vi "Cal Validation.vi"(0 "Path In":path, 5 "Probe Mic Gain (dB)":dbl, 7 "Cal Mic Gain (dB)":dbl, 9 "Cal Mic Sens (dB)":dbl, 11 "Ear":T2) -> ()   [LabVIEW 2020]
uses:
  Utility VIs/Type Defs/Left-Right ring.ctl
  Type Defs/Cal-Smoothing Parameters.ctl
  Type Defs/CalVal-Params.ctl
panel:
  out "Smooth Params":T1={"Method"=enum."Loess", "MA"={"Iterations"=100, "Length"=3}, "Loess"={"Length"=21, "Type"=enum."Quadratic", "Robust"=TRUE}} {"Loess"."Length" min=1 step=1; "MA"."Length" min=1 step=1; "MA"."Iterations" min=1 step=1}
  in  "Save Button":bool
  out "df (Hz)":dbl
  out "Fs (Hz)":dbl
  out "Frequency (Hz)":dbl
  out "Test Freqs":dbl[](array[numeric])
  out "Error Graph":T3(graph)
  out "Mag Graph":T3(graph)
  out "exit signal":bool
  out "Path":path
  out "running":bool
  in  "Exit":bool
  in  "Go":bool
  out "Abort":bool
  in  "Stop":bool
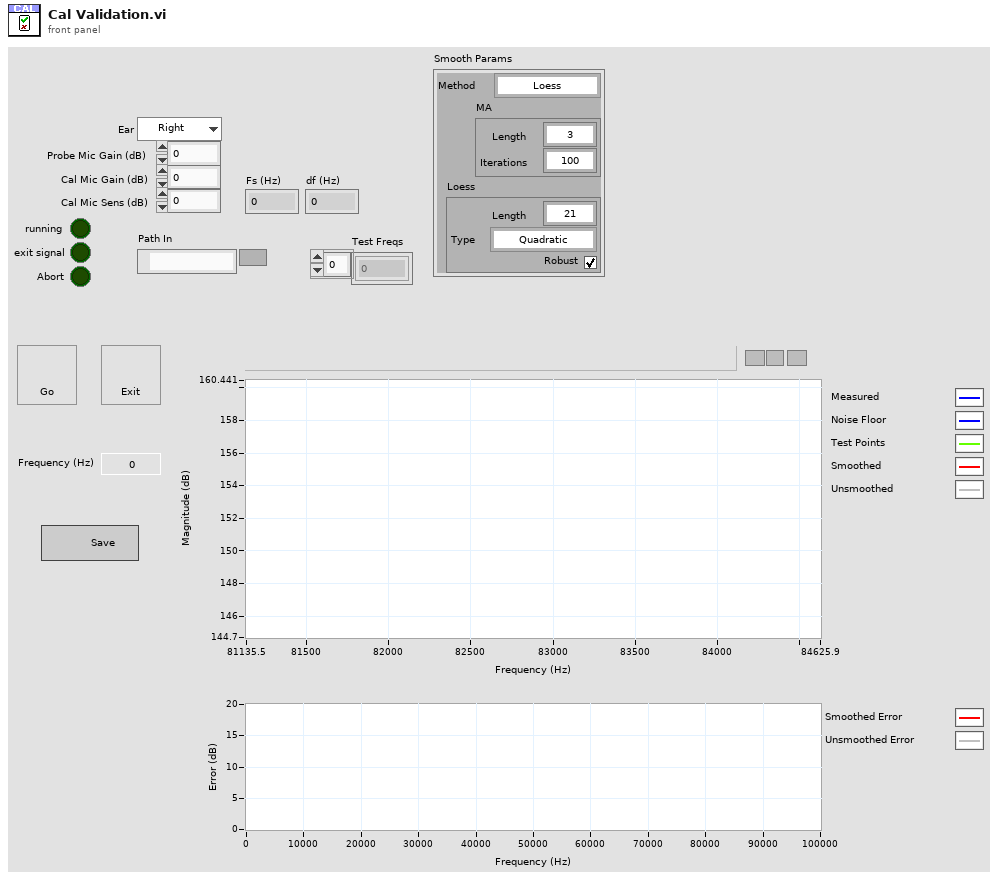
[diagram p1: front panel]
types:
  T1 = typedef "Cal-Smoothing Parameters.ctl" = cluster{"Method":enum16{"None", "Moving average", "Loess"}, "MA":cluster{"Iterations":i32, "Length":i32}, "Loess":cluster{"Length":i32, "Type":enum16{"Linear", "Quadratic"}, "Robust":bool}}
  T2 = typedef "Left-Right ring.ctl" = enum16{"Right", "Left"}
  T3 = cluster{"Frequency (Hz)":dbl[], "Unsmoothed Mag":dbl[]}[]
  T4 = cluster{"Freq (Hz)":dbl, "Val (dB SPL/V)":dbl, "Noise Floor":dbl}
  T5 = typedef "CalVal-Params.ctl" = cluster{"Fs (Hz)":dbl, "Duration (s)":dbl, "Ear":T2, "Probe Mic Gain (dB)":dbl, "Cal Mic Gain (dB)":dbl, "Cal Mic Sens (dB)":dbl, "AO Channels":i32[], "NPts/buffer":i32, "Probe-Cal Indices":i32[]}
  T6 = enum8{"Enabled", "Disabled", "Disabled and Grayed Out"}
  T7 = cluster{"Frequency (Hz)":dbl[], "Unsmoothed Mag":dbl[]}
  T8 = cluster{"Length":i32, "Type":enum16{"Linear", "Quadratic"}, "Robust":bool}
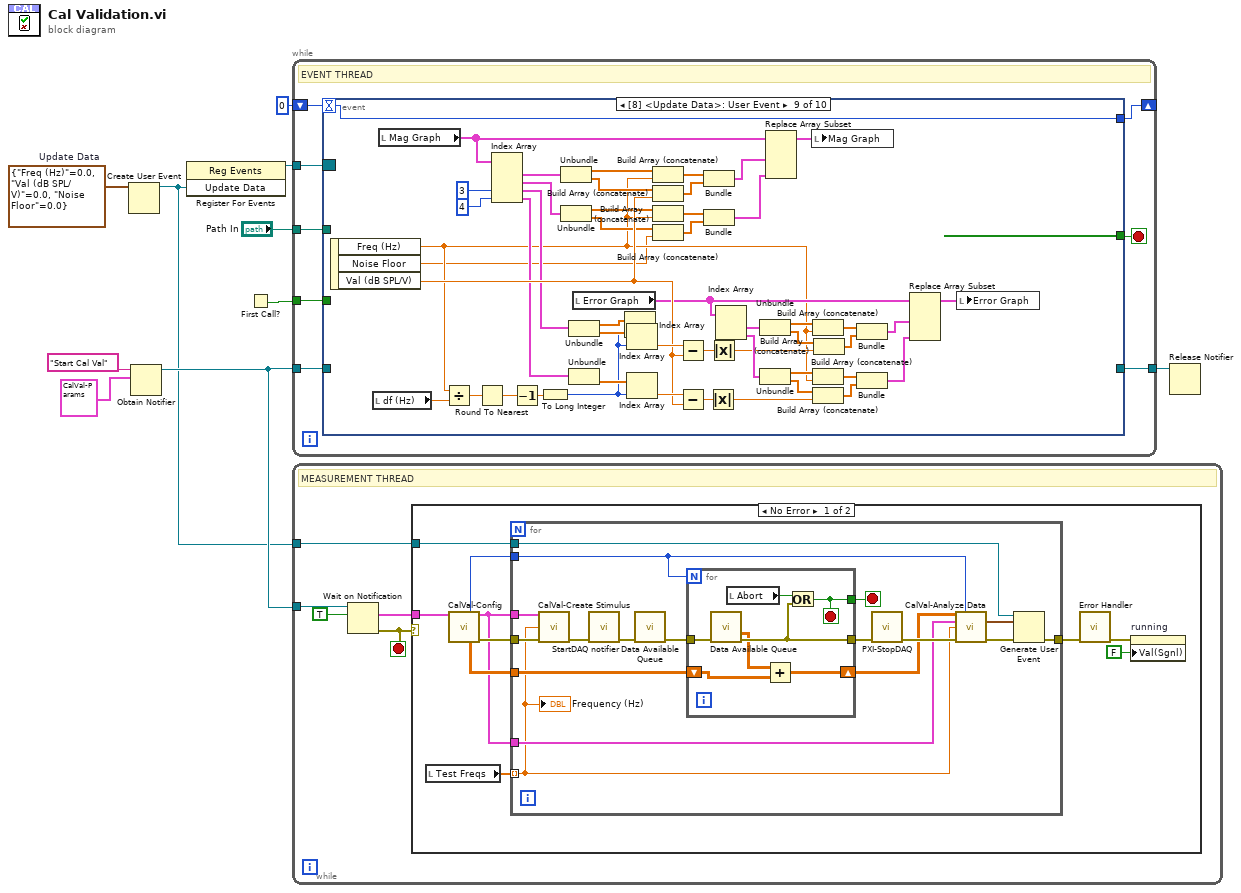
[diagram p0: block diagram]
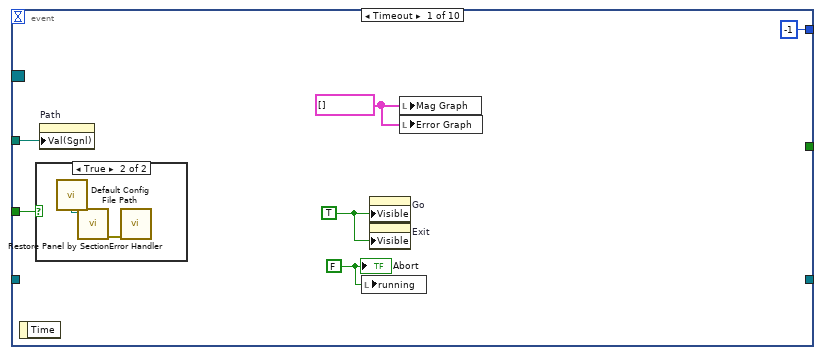
[diagram p3: hidden frame]
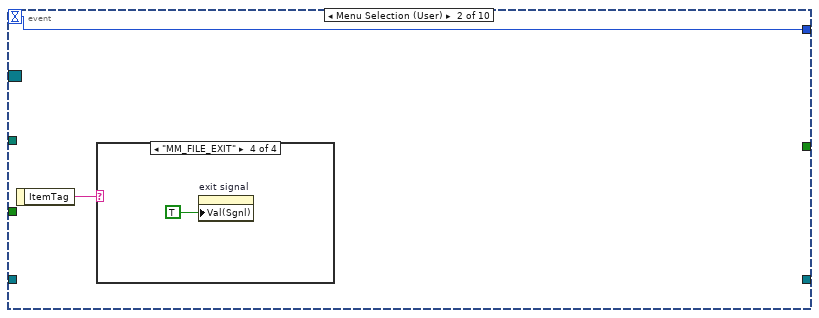
[diagram p5: hidden frame]
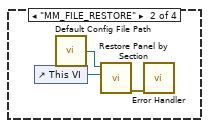
[diagram p7: hidden frame]
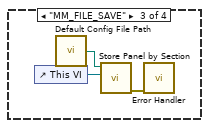
[diagram p8: hidden frame]
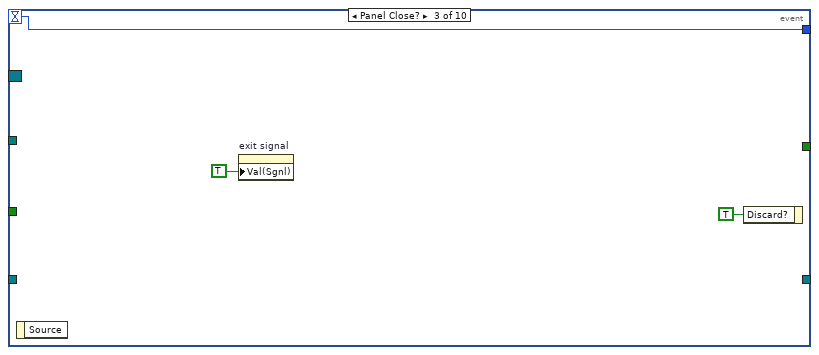
[diagram p9: hidden frame]
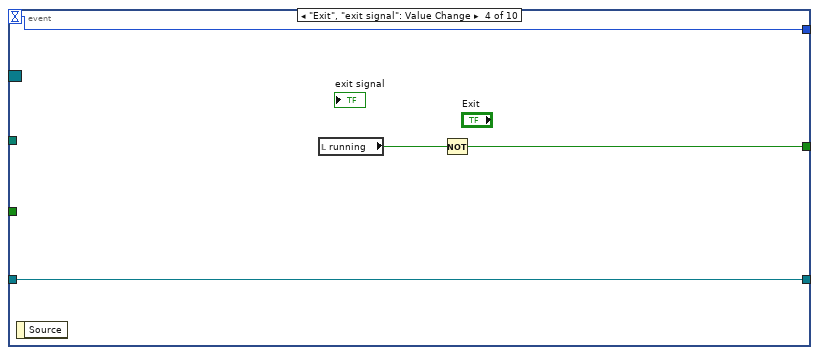
[diagram p10: hidden frame]
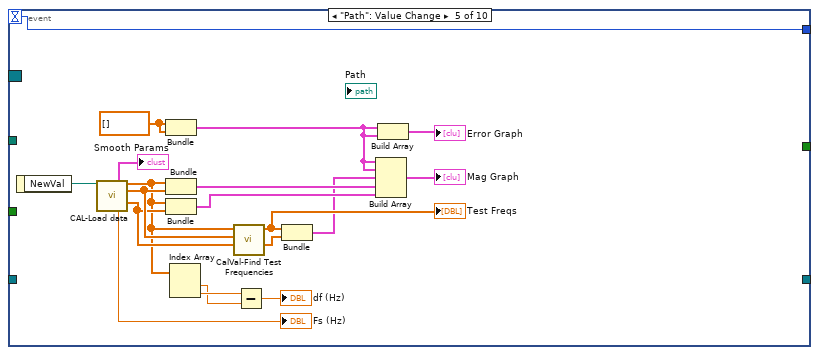
[diagram p11: hidden frame]
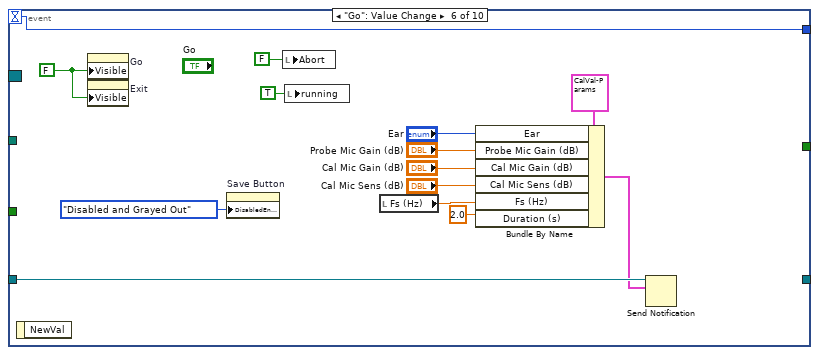
[diagram p12: hidden frame]
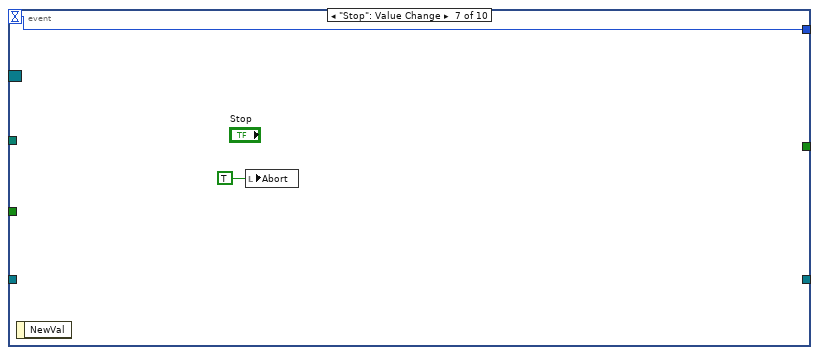
[diagram p13: hidden frame]
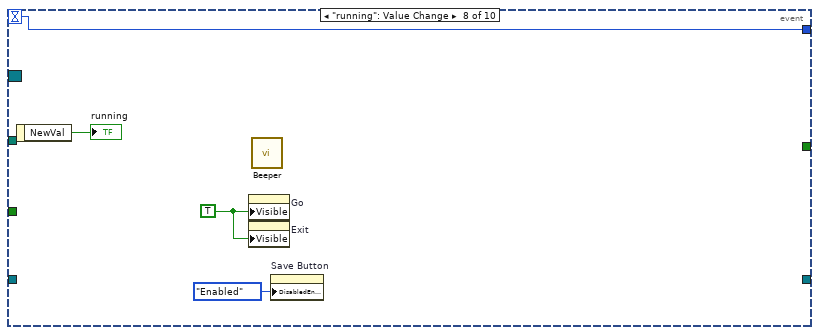
[diagram p14: hidden frame]
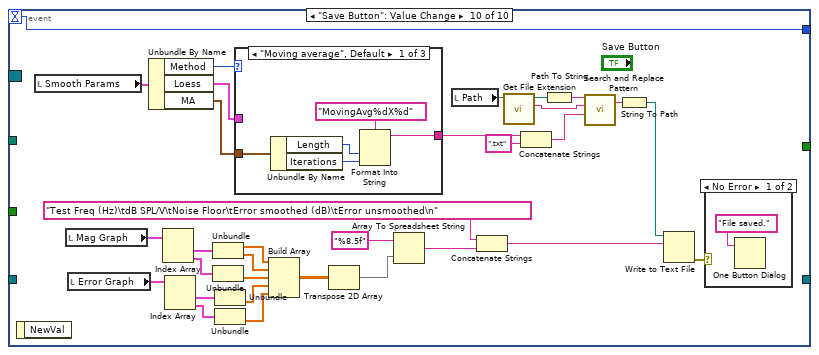
[diagram p15: hidden frame]
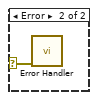
[diagram p16: hidden frame]
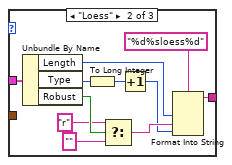
[diagram p17: hidden frame]
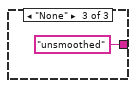
[diagram p18: hidden frame]
diagram:
  w2 = T4 {"Freq (Hz)"=0.0, "Val (dB SPL/V)"=0.0, "Noise Floor"=0.0}  # Update Data
  n1 = Create User Event(user event datatype=w2) -> (user event=w1:refnum<user-event>)  [unwired: 1 in, 1 out]
  n2 = Obtain Notifier(name (unnamed)="Start Cal Val", notification data type=T5 {"Fs (Hz)"=0.0, "Duration (s)"=0.0, "Ear"=enum."Right", "Probe Mic Gain (dB)"=0.0, "Cal Mic Gain (dB)"=0.0, "Cal Mic Sens (dB)"=0.0, "AO Channels"=[], "NPts/buffer"=0, "Probe-Cal Indices"=[]} ("Params")) -> (notifier out=w10:refnum<notifier>)  [unwired: 2 in, 2 out]
  n3 = register-events(w1) -> (reference out=w3:refnum<event-registration>)  [unwired: 2 in, 1 out]
  n4 = First Call?() -> (First Call?: T/F=w6:bool)
  n5 = while {
    tunnel: w10 -> [w18]
    tunnel: [w16] -> w9
    shift-right: [w14] -> _
    shift-left: 0 -> [w15]
    tunnel: w6 -> [w13]
    tunnel: "Path In" -> [w12]
    tunnel: w3 -> [w11]
    stop <- w17 stop-if-true
    # "EVENT THREAD"
    n6 = event shown="[8] <Update Data>: User Event" {
      selector: w11 -> [_ _ _ _ _ _ _ _ _ _]
      dyn-events: _ -> [_ _ _ _ _ _ _ _ _ _]
      timeout: w15 -> [_ w27 w38 w41 w61 w73 w76 w81 w131 w163]
      tunnel: w18 -> [_ _ _ w42 _ w75 _ _ _ _]
      tunnel: [_ _ _ w39 _ _ _ _ _ _] -> w17
      tunnel: [_ _ _ w42 _ _ _ _ _ _] -> w16
      tunnel: [-1 w27 w38 w41 w61 w73 w76 w81 w131 w163] -> w14
      tunnel: w13 -> [w22 _ _ _ _ _ _ _ _ _]
      tunnel: w12 -> [w19 _ _ _ _ _ _ _ _ _]
      event Timeout {
        w20 = T3 [] ("Mag Graph")
        w21 = TRUE ("Visible")
        w23 = FALSE ("Abort")
        n7 = event-data() -> ()  [unwired: 1 in, 1 out]
        n8 = case shown="True" w22 {
          frame False {
          }
          frame True {
            n9 = call "Default Config File Path.vi"() -> ("Default config file name"=w25:path)
            n10 = call "Restore Panel by Section.vi"("Path (dialog)"=w25) -> ("Error Out"=w26:errorcluster)  [unwired: 10 in]
            n11 = call "Error Handler.vi"("error in (no error)"=w26) -> ()  [unwired: 13 in, 2 out]
          }
        }
        n12 = property on="Path" class="Path"("Val(Sgnl)"=w19) -> ()  [unwired: 2 in, 2 out]
        n13 = local write "running"(w23) -> ()
        n14 = property on="Go" class="Bool"("Visible"=w21) -> ()  [unwired: 2 in, 2 out]
        n15 = property on="Exit" class="Bool"("Visible"=w21) -> ()  [unwired: 2 in, 2 out]
        n16 = local write "Mag Graph"(w20) -> ()
        n17 = local write "Error Graph"(w20) -> ()
        "Abort" <- w23
      }
      event Menu Selection (User) {
        n18 = event-data() -> ("ItemTag"=w28:string)  [unwired: 1 in]
        n19 = case shown="\"MM_FILE_EXIT\"" w28 {
          frame "False", Default {
          }
          frame "MM_FILE_RESTORE" {
            n20 = control-ref of="This VI"() -> (w30:refnum<vi>)
            n21 = call "Default Config File Path.vi"() -> ("Default config file name"=w29:path)
            n22 = call "Restore Panel by Section.vi"("VI reference"=w30, "Path (dialog)"=w29) -> ("Error Out"=w31:errorcluster)  [unwired: 9 in]
            n23 = call "Error Handler.vi"("error in (no error)"=w31) -> ()  [unwired: 13 in, 2 out]
          }
          frame "MM_FILE_SAVE" {
            n24 = control-ref of="This VI"() -> (w33:refnum<vi>)
            n25 = call "Default Config File Path.vi"() -> ("Default config file name"=w32:path)
            n26 = call "Store Panel by Section.vi"("VI reference"=w33, "Path (dialog)"=w32) -> ("Error Out"=w34:errorcluster)  [unwired: 9 in]
            n27 = call "Error Handler.vi"("error in (no error)"=w34) -> ()  [unwired: 13 in, 2 out]
          }
          frame "MM_FILE_EXIT" {
            n28 = property on="exit signal" class="Bool (strict)"("Val(Sgnl)"=TRUE ("Value (Signaling)")) -> ()  [unwired: 2 in, 2 out]
          }
        }
      }
      event Panel Close? {
        n29 = event-data() -> ()  [unwired: 1 in, 1 out]
        n30 = property on="exit signal" class="Bool (strict)"("Val(Sgnl)"=TRUE ("Value (Signaling)")) -> ()  [unwired: 2 in, 2 out]
        n31 = event-data("Discard?"=TRUE) -> ()  [unwired: 1 in, 1 out]
      }
      event "Exit", "exit signal": Value Change {
        n32 = event-data() -> ()  [unwired: 1 in, 1 out]
        n33 = local read "running"() -> (w40:bool)
        n34 = Not(x=w40) -> (.not. x?=w39:bool)
      }
      event "Path": Value Change {
        w57 = dbl[] []
        n35 = event-data() -> ("NewVal"=w60:path)  [unwired: 1 in]
        n36 = call "CAL-Load data.vi"("user path"=w60) -> ("Smooth Params"=→"Smooth Params":T1, "Frequency (Hz)"=w46:dbl[], "Mag"=w56:dbl[], "Unsmoothed Mag"=w55:dbl[], "Fs (Hz)"=→"Fs (Hz)":dbl)  [unwired: 7 in, 3 out]
        n37 = Bundle(w57, w57) -> (w48:cluster{dbl[], dbl[]})  [unwired: 1 in]
        n38 = Bundle("Frequency (Hz)"=w46, "Mag"=w56) -> (w59:cluster{"Frequency (Hz)":dbl[], "Mag":dbl[]})  [unwired: 1 in]
        n39 = Bundle("Frequency (Hz)"=w46, "Unsmoothed Mag"=w55) -> (w58:T7)  [unwired: 1 in]
        n40 = Index Array(array=w46) -> (element #1=w44:dbl, element #2=w45:dbl)  [unwired: 2 in]
        n41 = call "CalVal-Find Test Frequencies.vi"("Unsmoothed"=w55, "Smoothed"=w56, "Frequency"=w46) -> ("Mags"=w52:dbl[], "Test Freqs"=w53:dbl[])  [unwired: 7 in]
        "Test Freqs" <- w53
        n42 = Subtract(x=w45, y=w44) -> (x-y=→"df (Hz)":dbl)
        n43 = Bundle("Test Freqs"=w53, "Mags"=w52) -> (w51:cluster{"Test Freqs":dbl[], "Mags":dbl[]})  [unwired: 1 in]
        n44 = Build Array(w48, w48, w51, w59, w58) -> (→"Mag Graph":T3)
        n45 = Build Array(w48, w48) -> (→"Error Graph":cluster{dbl[], dbl[]}[])
      }
      event "Go": Value Change {
        w72 = FALSE ("Visible")
        n46 = event-data() -> ()  [unwired: 1 in, 1 out]
        n47 = property on="Go" class="Bool"("Visible"=w72) -> ()  [unwired: 2 in, 2 out]
        n48 = property on="Exit" class="Bool"("Visible"=w72) -> ()  [unwired: 2 in, 2 out]
        n49 = property on="Save Button" class="Bool"("DisabledEnum"=T6."Disabled and Grayed Out" ("Disabled")) -> ()  [unwired: 2 in, 2 out]
        n50 = local write "Abort"(FALSE ("Abort")) -> ()
        n51 = local write "running"(TRUE ("running")) -> ()
        n52 = local read "Fs (Hz)"() -> (w63:dbl)
        n53 = Bundle By Name(cluster=T5 {"Fs (Hz)"=0.0, "Duration (s)"=0.0, "Ear"=enum."Right", "Probe Mic Gain (dB)"=0.0, "Cal Mic Gain (dB)"=0.0, "Cal Mic Sens (dB)"=0.0, "AO Channels"=[], "NPts/buffer"=0, "Probe-Cal Indices"=[]} ("Params"), "Ear"="Ear", "Probe Mic Gain (dB)"="Probe Mic Gain (dB)", "Cal Mic Gain (dB)"="Cal Mic Gain (dB)", "Cal Mic Sens (dB)"="Cal Mic Sens (dB)", "Fs (Hz)"=w63, "Duration (s)"=2.0) -> (w69:T5)
        n54 = Send Notification(notification=w69, notifier=w75) -> ()  [unwired: 1 in, 2 out]
      }
      event "Stop": Value Change {
        n55 = event-data() -> ()  [unwired: 1 in, 1 out]
        n56 = local write "Abort"(TRUE ("Abort")) -> ()
      }
      event "running": Value Change {
        w80 = TRUE ("Visible")
        n57 = event-data() -> ("NewVal"=→"running":bool)  [unwired: 1 in]
        n58 = property on="Go" class="Bool"("Visible"=w80) -> ()  [unwired: 2 in, 2 out]
        n59 = property on="Exit" class="Bool"("Visible"=w80) -> ()  [unwired: 2 in, 2 out]
        n60 = call "Beeper.vi"() -> ()  [unwired: 5 in, 1 out]
        n61 = property on="Save Button" class="Bool"("DisabledEnum"=T6."Enabled" ("Disabled")) -> ()  [unwired: 2 in, 2 out]
      }
      event User Event {
        n62 = event-data() -> ("Freq (Hz)"=w88:dbl, "Noise Floor"=w87:dbl, "Val (dB SPL/V)"=w117:dbl)  [unwired: 1 in]
        n63 = local read "df (Hz)"() -> (w86:dbl)
        n64 = local read "Mag Graph"() -> (w125:T3)
        n65 = Divide(x=w88, y=w86) -> (x/y=w122:dbl)
        n66 = Round To Nearest(number=w122) -> (nearest integer value=w85:dbl)
        n67 = Index Array(array=w125, index #3=3 ("index"), index #4=4 ("index")) -> (element #1=w130:T7, element #2=w90:T7, element #3=w95:T7, element #4=w96:T7)  [unwired: 2 in]
        n68 = Decrement(x=w85) -> (x-1=w84:dbl)
        n69 = To Long Integer(number=w84) -> (32bit integer=w82:i32)
        n70 = Unbundle(w130) -> ("Frequency (Hz)"=w129:dbl[], "Unsmoothed Mag"=w128:dbl[])
        n71 = Unbundle(w90) -> ("Frequency (Hz)"=w94:dbl[], "Unsmoothed Mag"=w93:dbl[])
        n72 = Unbundle(w95) -> ("Frequency (Hz)"=w83:dbl[], "Unsmoothed Mag"=w121:dbl[])
        n73 = Unbundle(w96) -> ("Unsmoothed Mag"=w120:dbl[])  [unwired: 1 out]
        n74 = local read "Error Graph"() -> (w115:T3)
        n75 = Index Array(array=w83, index=w82) -> ()  [unwired: 1 out]
        n76 = Index Array(array=w121, index=w82) -> (element=w118:dbl)
        n77 = Index Array(array=w120, index=w82) -> (element=w119:dbl)
        n78 = Build Array (concatenate)(w129, w88) -> (w127:dbl[])
        n79 = Build Array (concatenate)(w128, w117) -> (w126:dbl[])
        n80 = Build Array (concatenate)(w94, w88) -> (w92:dbl[])
        n81 = Build Array (concatenate)(w93, w87) -> (w91:dbl[])
        n82 = Subtract(x=w118, y=w117) -> (x-y=w102:dbl)
        n83 = Subtract(x=w119, y=w117) -> (x-y=w101:dbl)
        n84 = Bundle(w127, w126) -> (w124:cluster{dbl[], dbl[]})  [unwired: 1 in]
        n85 = Bundle(w92, w91) -> (w89:cluster{dbl[], dbl[]})  [unwired: 1 in]
        n86 = Absolute Value(x=w101) -> (abs(x)=w99:dbl)
        n87 = Absolute Value(x=w102) -> (abs(x)=w100:dbl)
        n88 = Index Array(array=w115) -> (element #1=w108:T7, element #2=w113:T7)  [unwired: 2 in]
        n89 = Unbundle(w108) -> ("Frequency (Hz)"=w107:dbl[], "Unsmoothed Mag"=w106:dbl[])
        n90 = Unbundle(w113) -> ("Frequency (Hz)"=w112:dbl[], "Unsmoothed Mag"=w111:dbl[])
        n91 = Replace Array Subset(array=w125, new element #1=w124, new element #2=w89) -> (w123:T3)  [unwired: 2 in]
        n92 = local write "Mag Graph"(w123) -> ()
        n93 = Build Array (concatenate)(w107, w88) -> (w105:dbl[])
        n94 = Build Array (concatenate)(w112, w88) -> (w110:dbl[])
        n95 = Build Array (concatenate)(w111, w99) -> (w109:dbl[])
        n96 = Build Array (concatenate)(w106, w100) -> (w104:dbl[])
        n97 = Bundle(w105, w104) -> (w103:cluster{dbl[], dbl[]})  [unwired: 1 in]
        n98 = Bundle(w110, w109) -> (w114:cluster{dbl[], dbl[]})  [unwired: 1 in]
        n99 = Replace Array Subset(array=w115, new element #1=w103, new element #2=w114) -> (w116:T3)  [unwired: 2 in]
        n100 = local write "Error Graph"(w116) -> ()
      }
      event "Save Button": Value Change {
        n101 = event-data() -> ()  [unwired: 1 in, 1 out]
        n102 = local read "Smooth Params"() -> (w147:T1)
        n103 = local read "Mag Graph"() -> (w161:T3)
        n104 = local read "Error Graph"() -> (w162:T3)
        n105 = Unbundle By Name(w147) -> ("Method"=w146:enum16{"None", "Moving average", "Loess"}, "Loess"=w144:T8, "MA"=w145:cluster{"Iterations":i32, "Length":i32})
        n106 = Index Array(array=w161) -> (element #1=w160:T7, element #2=w133:T7)  [unwired: 2 in]
        n107 = Index Array(array=w162) -> (element #1=w159:T7, element #2=w158:T7)  [unwired: 2 in]
        n108 = Unbundle(w160) -> ("Frequency (Hz)"=w157:dbl[], "Unsmoothed Mag"=w156:dbl[])
        n109 = Unbundle(w133) -> ("Unsmoothed Mag"=w132:dbl[])  [unwired: 1 out]
        n110 = Unbundle(w159) -> ("Unsmoothed Mag"=w155:dbl[])  [unwired: 1 out]
        n111 = Unbundle(w158) -> ("Unsmoothed Mag"=w154:dbl[])  [unwired: 1 out]
        n112 = case shown="\"Moving average\", Default" w146 {
          tunnel: w144 -> [_ w180 _]
          tunnel: w145 -> [w170 _ _]
          tunnel: [w168 w178 "unsmoothed"] -> w140
          frame "Moving average", Default {
            n113 = Unbundle By Name(w170) -> ("Length"=w167:i32, "Iterations"=w166:i32)
            n114 = Format Into String(format string="MovingAvg%dX%d", w167, w166) -> (resulting string=w168:string)  [unwired: 2 in, 1 out]
          }
          frame "Loess" {
            n115 = Unbundle By Name(w180) -> ("Length"=w177:i32, "Type"=w181:enum16{"Linear", "Quadratic"}, "Robust"=w175:bool)
            n116 = To Long Integer(number=w181) -> (32bit integer=w176:i32)
            n117 = Select(t="r", s=w175, f="") -> (s? t:f=w172:string)
            n118 = Increment(x=w176) -> (x+1=w171:i32)
            n119 = Format Into String(format string="%d%sloess%d", w177, w172, w171) -> (resulting string=w178:string)  [unwired: 2 in, 1 out]
          }
          frame "None" {
          }
        }
        n120 = Build Array(w157, w156, w132, w155, w154) -> (w152:dbl[][])
        n121 = Transpose 2D Array(2D array=w152) -> (transposed array=w151:dbl[][])
        n122 = Array To Spreadsheet String(array=w151, 3:"%8.5f" ("format (%.3f)")) -> (spreadsheet string=w150:string)  [unwired: 1 in]
        n123 = local read "Path"() -> (w143:path)
        n124 = Concatenate Strings("Test Freq (Hz)\tdB SPL/V\tNoise Floor\tError smoothed (dB)\tError unsmoothed\n" ("string"), w150) -> (w148:string)
        n125 = call <vilib>:"Get File Extension.vi"("file"=w143) -> ("lowercase file extension"=w139:string, "dup file"=w142:path)  [unwired: 6 in, 3 out]
        n126 = Concatenate Strings(w140, ".txt" ("string")) -> (w138:string)
        n127 = Path To String(path=w142) -> (string=w141:string)
        n128 = call <vilib>:"Search and Replace Pattern.vi"("string"=w141, "regular expression (\"\")"=w139, "replace string (\"\")"=w138) -> ("result string"=w137:string)  [unwired: 2 in, 1 out]
        n129 = String To Path(string=w137) -> (path=w136:path)
        n130 = Write to Text File(file (use dialog)=w136, text=w148) -> (error out=w134:errorcluster)  [unwired: 2 in, 2 out]
        n131 = case shown="No Error" w134 {
          selector: w134 -> [_ w165]
          frame No Error {
            n132 = One Button Dialog(message="File saved.") -> ()  [unwired: 1 in, 1 out]
          }
          frame Error {
            n133 = call "Error Handler.vi"("error in (no error)"=w165) -> ()  [unwired: 13 in, 2 out]
          }
        }
      }
    }
  }
  n134 = while {
    tunnel: w10 -> [w186]
    tunnel: w1 -> [w183]
    stop <- w184 stop-if-true
    # "MEASUREMENT THREAD"
    n135 = Wait on Notification(notifier=w186, ignore previous (F)=TRUE) -> (notification=w185:T5, error out=w184:errorcluster)  [unwired: 2 in, 2 out]
    n136 = case shown="No Error" w184 {
      tunnel: w185 -> [w196 _]
      tunnel: w183 -> [w189 _]
      frame No Error {
        n137 = local read "Test Freqs"() -> (w188:dbl[])
        n138 = call "CalVal-Config.vi"("Params In"=w196) -> ("NBuffers"=w193:i32, "Params Out"=w190:T5, "Mic Avg"=w195:dbl[][], "error out"=w194:errorcluster)  [unwired: 11 in]
        n139 = for {
          tunnel: w188 -> [w199] mode=indexing
          tunnel: w190 -> [w211]
          tunnel: w195 -> [w213]
          tunnel: w194 -> [w214]
          tunnel: w193 -> [w203]
          tunnel: [w200] -> w191
          tunnel: w190 -> [w205]
          tunnel: w189 -> [w202]
          stop <- w208 stop-if-true
          n140 = call "CalVal-Create Stimulus.vi"("Params"=w211, "Test Freq (Hz)"=w199, "error in (no error)"=w214) -> ("error out"=w212:errorcluster)  [unwired: 12 in]
          n141 = call "StartDAQ notifier.vi"("error in (no error)"=w212) -> ("error out"=w210:errorcluster)  [unwired: 6 in]
          n142 = call "Data Available Queue.vi"("error in (no error)"=w210) -> ("error out"=w209:errorcluster)  [unwired: 10 in, 4 out]
          n143 = for {
            N: w203 -> [_]
            tunnel: w209 -> [w220]
            shift-right: [w215] -> w204
            shift-left: w213 -> [w216]
            tunnel: [w219] -> w207
            tunnel: [w218] -> w208
            stop <- w218 stop-if-true
            n144 = call "Data Available Queue.vi"("error in (no error)"=w220) -> ("AI Waveforms"=w217:dbl[][], "error out"=w219:errorcluster)  [unwired: 10 in, 3 out]
            n145 = local read "Abort"() -> (w221:bool)
            n146 = Add(x=w217, y=w216) -> (x+y=w215:dbl[][])
            n147 = Or(x=w221, y=w219) -> (x .or. y?=w218:bool)
          }
          n148 = call "PXI-StopDAQ.vi"("error in (no error)"=w207) -> ("error out"=w206:errorcluster)  [unwired: 6 in]
          n149 = call "CalVal-Analyze Data.vi"("Data"=w204, "Navgs"=w203, "Params"=w205, "Test Freq (Hz)"=w199, "error in (no error)"=w206) -> ("Update Data"=w198:T4, "error out"=w201:errorcluster)  [unwired: 9 in]
          n150 = Generate User Event(user event=w202, event data cluster=w198, error in=w201) -> (error out=w200:errorcluster)  [unwired: 1 in, 1 out]
          "Frequency (Hz)" <- w199
        }
        n151 = call "Error Handler.vi"("error in (no error)"=w191) -> ("No Error"=w192:errorcluster)  [unwired: 13 in, 1 out]
        n152 = property on="running" class="Bool (strict)"(error in=w192, "Val(Sgnl)"=FALSE ("Value (Signaling)")) -> ()  [unwired: 1 in, 2 out]
      }
      frame Error {
      }
    }
  }
  n153 = Release Notifier(notifier=w9) -> ()  [unwired: 2 in, 3 out]
